vi "Attribute Array to Cluster.vi"(5 "Cluster Type":variant, 6 "error in (no error)":errorcluster, 7 "Values":variant[](array[variant]), 8 "Names":string[](array[string])) -> (0 "error out":errorcluster, 3 "Cluster":variant)   [LabVIEW 2017]
doc: "Converts a cluster to arrays of element names and element values"
panel:
  # "LVHDF5 Toolkit\nCopyright (c) 2005-2013 by Jason D. Sommerville\nCopyright (c) 2014 by UPVI, LLC.\n\nThis use and distribution of this file is governed by the terms found in \nLICENSE.txt distributed with this toolkit and installed at\n <user.lib>\\_lvhdf5\\LICENSE.txt"
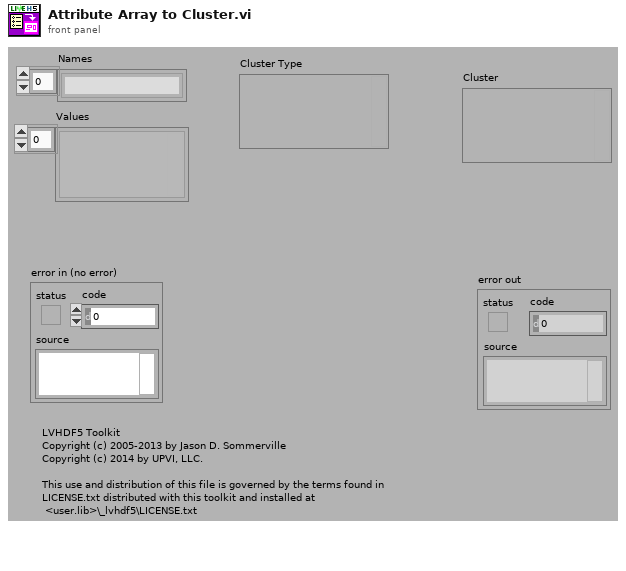
[diagram p1: front panel]
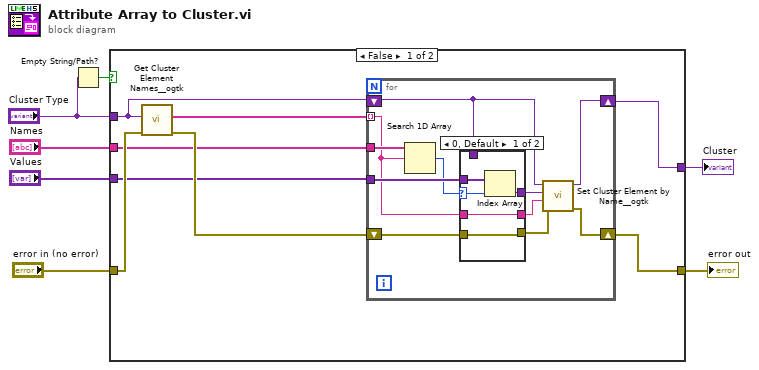
[diagram p0: block diagram]
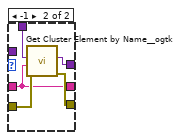
[diagram p2: hidden frame]
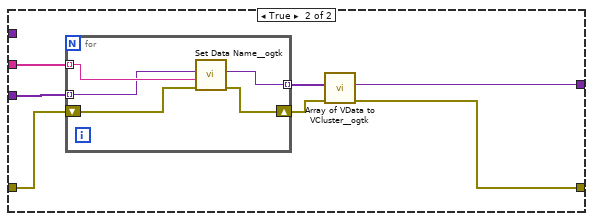
[diagram p3: hidden frame]
diagram:
  n1 = Empty String/Path?(string/path="Cluster Type") -> (empty?=w6:bool)
  n2 = case shown="False" w6 {
    tunnel: "Cluster Type" -> [w13 _]
    tunnel: "error in (no error)" -> [w15 w42]
    tunnel: [w11 w40] -> w4
    tunnel: [w10 w39] -> w3
    tunnel: "Names" -> [w9 w38]
    tunnel: "Values" -> [w8 w37]
    frame False {
      n3 = call <userlib>:"Get Cluster Element Names__ogtk.vi"("error in (no error)"=w15, "Cluster"=w13) -> ("error out"=w12:errorcluster, "Element Names"=w14:string[])  [unwired: 8 in]
      n4 = for {
        tunnel: w9 -> [w26]
        tunnel: w14 -> [w19] mode=indexing
        tunnel: w8 -> [w25]
        shift-right: [w23] -> w10
        shift-left: w12 -> [w20]
        shift-right: [w22] -> w11
        shift-left: w13 -> [w16]
        n5 = Search 1D Array(1D array=w26, element=w19) -> (index of element=w21:i32)  [unwired: 1 in]
        n6 = case shown="0, Default" w21 {
          selector: w21 -> [w29 _]
          tunnel: w25 -> [w31 _]
          tunnel: [w30 w33] -> w24
          tunnel: w20 -> [w27 w36]
          tunnel: w19 -> [w28 w34]
          tunnel: [w27 w35] -> w18
          tunnel: [w28 w34] -> w17
          tunnel: w16 -> [_ w32]
          frame 0, Default {
            n7 = Index Array(array=w31, index=w29) -> (element=w30:variant)
          }
          frame -1 {
            n8 = call <userlib>:"Get Cluster Element by Name__ogtk.vi"("error in (no error)"=w36, "Element Name"=w34, "Cluster"=w32) -> ("error out"=w35:errorcluster, "VElement"=w33:variant)  [unwired: 6 in, 1 out]
          }
        }
        n9 = call <userlib>:"Set Cluster Element by Name__ogtk.vi"("error in (no error)"=w18, "Element Name (\"\": New Element Data Name)"=w17, "New Element Value"=w24, "Cluster"=w16) -> ("error out"=w23:errorcluster, "VCluster out"=w22:variant)  [unwired: 5 in, 1 out]
      }
    }
    frame True {
      n10 = for {
        tunnel: [w48] -> w43 mode=indexing
        shift-right: [w46] -> w41
        shift-left: w42 -> [w47]
        tunnel: w38 -> [w45] mode=indexing
        tunnel: w37 -> [w44] mode=indexing
        n11 = call <userlib>:"Set Data Name__ogtk.vi"("error in (no error)"=w47, "Data Name"=w45, "Data"=w44) -> ("error out"=w46:errorcluster, "Renamed Data"=w48:variant)  [unwired: 7 in]
      }
      n12 = call <userlib>:"Array of VData to VCluster__ogtk.vi"("error in (no error)"=w41, "Array"=w43) -> ("error out"=w39:errorcluster, "VCluster"=w40:variant)  [unwired: 8 in]
    }
  }
  "error out" <- w3
  "Cluster" <- w4
